vi "Force Offsets DAO.vi"(7 "Tag":string, 8 "error in (no error)":errorcluster, 9 "Offsets In":T1, 10 "LBCB Number":T2, 11 "DAO Actions":T3) -> (0 "error out":errorcluster, 1 "Offsets Out":T1, 4 "Tags":string[](array[string]))   [LabVIEW 2009]
uses:
  Data Access Objects/Metadata/DAO Actions.ctl
  Data Access Objects/Metadata/LBCB Number.ctl
  Data Access Objects/Metadata/Actuator Point.ctl
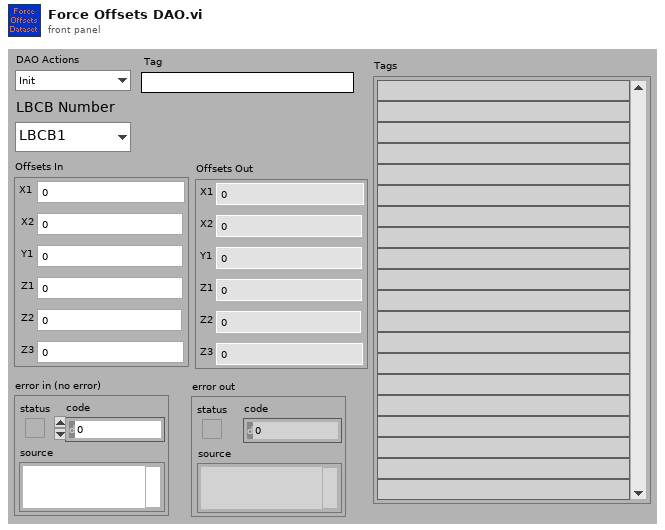
[diagram p1: front panel]
types:
  T1 = typedef "Actuator Point.ctl" = cluster{"X1":dbl, "X2":dbl, "Y1":dbl, "Z1":dbl, "Z2":dbl, "Z3":dbl}
  T2 = typedef "LBCB Number.ctl" = enum16{"LBCB1", "LBCB2"}
  T3 = typedef "DAO Actions.ctl" = enum16{"Init", "Get", "Set"}
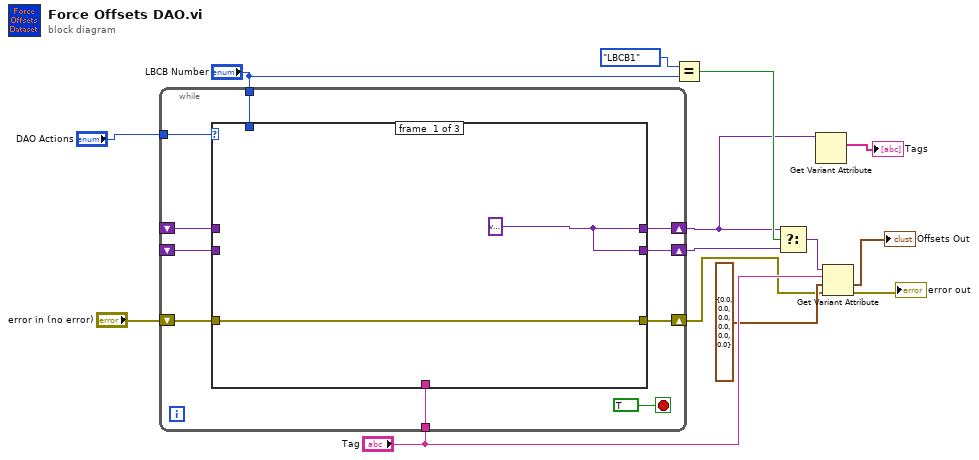
[diagram p0: block diagram]
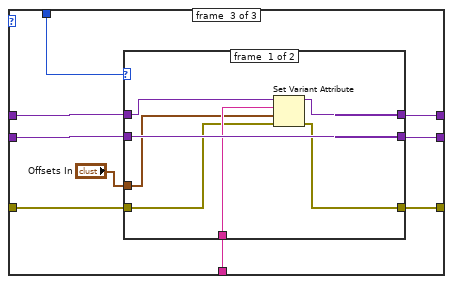
[diagram p3: hidden frame]
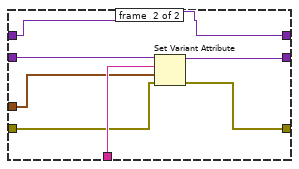
[diagram p4: hidden frame]
diagram:
  n1 = while {
    tunnel: "DAO Actions" -> [w23]
    shift-right: [w22] -> w2
    shift-left: _ -> [w19]
    tunnel: "LBCB Number" -> [w21]
    shift-right: [w20] -> w13
    shift-left: _ -> [w18]
    tunnel: "Tag" -> [w17]
    shift-right: [w15] -> w4
    shift-left: "error in (no error)" -> [w16]
    stop <- TRUE stop-if-true
    n2 = case shown="\"Set\"" w23 {
      tunnel: [w26 w29 w34] -> w22
      tunnel: w21 -> [_ _ w38]
      tunnel: [w26 w28 w36] -> w20
      tunnel: w19 -> [_ w29 w35]
      tunnel: w18 -> [_ w28 w33]
      tunnel: w17 -> [_ _ w32]
      tunnel: w16 -> [w25 w27 w31]
      tunnel: [w25 w27 w30] -> w15
      frame #0 {
        w26 = variant
      }
      frame #1 {
      }
      frame #2 {
        n3 = case shown="\"LBCB1\"" w38 {
          tunnel: "Offsets In" -> [w41 w51]
          tunnel: [w45 w48] -> w36
          tunnel: w35 -> [w44 w50]
          tunnel: [w43 w50] -> w34
          tunnel: w33 -> [w45 w49]
          tunnel: w32 -> [w42 w52]
          tunnel: w31 -> [w40 w47]
          tunnel: [w39 w46] -> w30
          frame #0 {
            n4 = Set Variant Attribute(Variant=w44, name=w42, value=w41, error in=w40) -> (Variant out=w43:variant, error out=w39:errorcluster)  [unwired: 1 out]
          }
          frame #1 {
            n5 = Set Variant Attribute(Variant=w49, name=w52, value=w51, error in=w47) -> (Variant out=w48:variant, error out=w46:errorcluster)  [unwired: 1 out]
          }
        }
      }
    }
  }
  n6 = Equal?(x=LBCB_Number."LBCB1", y="LBCB Number") -> (x = y?=w10:bool)
  n7 = Select(t=w2, s=w10, f=w13) -> (s? t:f=w8:variant)
  n8 = Get Variant Attribute(Variant=w2) -> (names=→"Tags":string[])  [unwired: 3 in, 3 out]
  n9 = Get Variant Attribute(Variant=w8, name="Tag", default value (empty Variant)=T1 {"X1"=0.0, "X2"=0.0, "Y1"=0.0, "Z1"=0.0, "Z2"=0.0, "Z3"=0.0} ("Offsets In"), error in=w4) -> (value=→"Offsets Out":T1, error out=→"error out":errorcluster)  [unwired: 2 out]
